vi "Msg To.vi"(9 "Queue Actor":refnum<class "Queue Actor.lvclass">, 10 "Alias":string) -> (3 "Queue Create Msg out":refnum<class "Queue Create Msg.lvclass">)   [LabVIEW 2021, in "jettl.lvlib" / "Queue Create.lvlib" / "Queue Create Msg.lvclass"]
uses:
  Queue Create Msg.lvclass
  jettl/Queue Actor/Queue Actor.lvclass
  Queue Create Msg.lvclass/Queue Create Msg.ctl
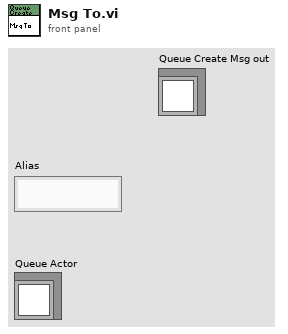
[diagram p1: front panel]
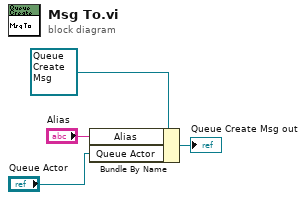
[diagram p0: block diagram]
diagram:
  n1 = Bundle By Name(cluster=refnum<class "Queue Create Msg.lvclass"> refnum ("Create Msg in"), "Alias"="Alias", "Queue Actor"="Queue Actor") -> (→"Queue Create Msg out":refnum<class "Queue Create Msg.lvclass">)
